vi "CreateFilePath_20210610.vi"(11 "base path":path=path "C:/Users/Bruce Wayne/Desktop/SourceCode_20171218/thresholds.csv") -> (0 "DateString":string, 1 "10 Hz appended path":path, 2 "appended path 2":path, 3 "appended path":path, 5 "Disdrom_Raw_String_File":path)   [LabVIEW 2018]
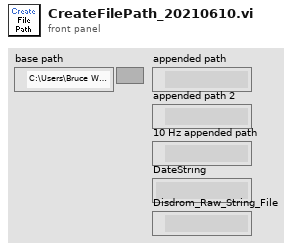
[diagram p1: front panel]
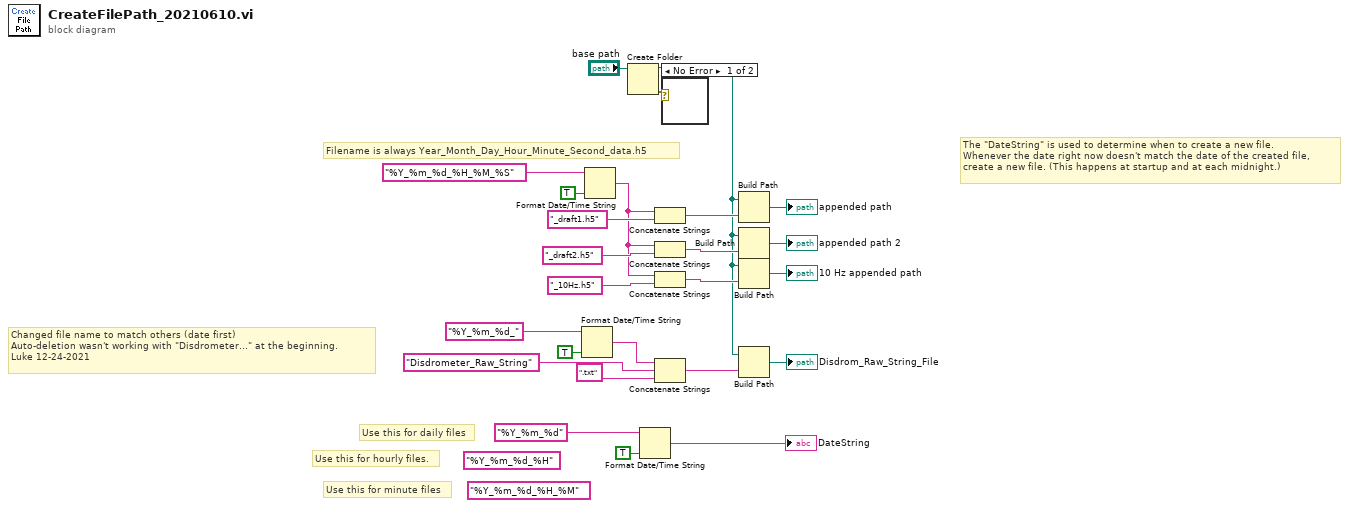
[diagram p0: block diagram]
diagram:
  (unwired) "%Y_%m_%d_%H" ("time format string (%c)")
  (unwired) "%Y_%m_%d_%H_%M" ("time format string (%c)")
  # "Changed file name to match others (date first)\nAuto-deletion wasn't working with \"Disdrometer...\" at the beginning.\nLuke 12-24-2021"
  # "Filename is always Year_Month_Day_Hour_Minute_Second_data.h5"
  # "The \"DateString\" is used to determine when to create a new file.\nWhenever the date right now doesn't match the date of the created file,\ncreate a new file. (This happens at startup and at each midnight.)"
  # "Use this for hourly files."
  # "Use this for daily files"
  # "Use this for minute files"
  n1 = Format Date/Time String(time format string (%c)="%Y_%m_%d_", UTC format=TRUE) -> (date/time string=w2:string)  [unwired: 1 in]
  n2 = Format Date/Time String(time format string (%c)="%Y_%m_%d_%H_%M_%S", UTC format=TRUE) -> (date/time string=w7:string)  [unwired: 1 in]
  n3 = Create Folder(path (use dialog)="base path") -> (created path=w3:path, error out=w23:errorcluster)  [unwired: 2 in, 1 out]
  n4 = Format Date/Time String(time format string (%c)="%Y_%m_%d", UTC format=TRUE) -> (date/time string=→"DateString":string)  [unwired: 1 in]
  n5 = Concatenate Strings(w7, "_draft1.h5" ("string")) -> (w21:string)
  n6 = Concatenate Strings(w7, "_draft2.h5" ("f")) -> (w14:string)
  n7 = Concatenate Strings(w7, "_10Hz.h5" ("f")) -> (w13:string)
  n8 = Concatenate Strings(w2, "Disdrometer_Raw_String" ("f"), ".txt" ("f")) -> (w8:string)
  n9 = case shown="No Error" w23 {
    frame No Error {
    }
    frame Error {
    }
  }
  n10 = Build Path(base path=w3, name or relative path=w21) -> (appended path=→"appended path":path)
  n11 = Build Path(base path=w3, name or relative path=w14) -> (appended path=→"appended path 2":path)
  n12 = Build Path(base path=w3, name or relative path=w13) -> (appended path=→"10 Hz appended path":path)
  n13 = Build Path(base path=w3, name or relative path=w8) -> (appended path=→"Disdrom_Raw_String_File":path)
